vi "solar Command.vi"(8 "error in (no error)":errorcluster, 9 "CMD_DATA":variant, 10 "CMD":string, 11 "solar in":refnum<class "solar.lvclass">) -> (0 "error out":errorcluster, 1 "TLM_DATA":variant, 2 "TLM":string, 3 "solar out":refnum<class "solar.lvclass">, 5 "Handled?":bool)   [LabVIEW 2018, in "solar.lvclass"]
doc: "Handles target commands."
uses:
  solar.lvclass
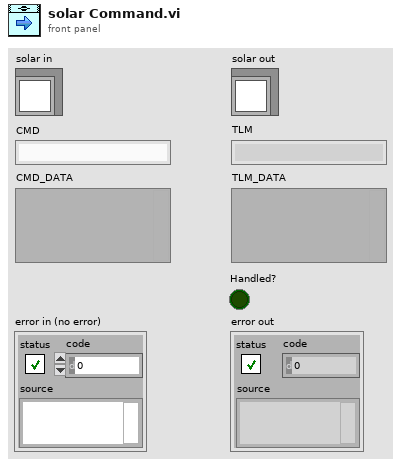
[diagram p1: front panel]
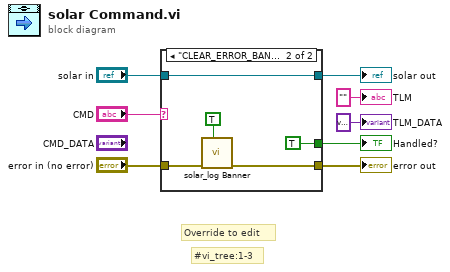
[diagram p0: block diagram]
diagram:
  # "#vi_tree:1-3"
  # "Override to edit"
  n1 = case shown="\"CLEAR_ERROR_BANNER\"" "CMD" {
    tunnel: "error in (no error)" -> [w9 w15]
    tunnel: [w9 w14] -> w5
    tunnel: "solar in" -> [w10 w12]
    tunnel: [w10 w12] -> w2
    tunnel: [_ TRUE] -> w1
    frame "False", Default {
    }
    frame "CLEAR_ERROR_BANNER" {
      n2 = call "solar_log Banner.vi"("Close? (F)"=TRUE, "error in (no error)"=w15) -> ("error out"=w14:errorcluster)  [unwired: 9 in]
    }
  }
  "error out" <- w5
  "solar out" <- w2
  "Handled?" <- w1
  "TLM" <- "" ("TLM_PACKET")
  "TLM_DATA" <- variant ("TLM_DATA")
